vi "max XY speed.vi"() -> ()   [LabVIEW 2018]
uses:
  Classes/Controller/Controller.lvclass
  Drivers/Aerotech A3200/Aerotech.lvlib
panel:
  in  "stop":bool
  out "Y max speed":dbl
  out "X max speed":dbl
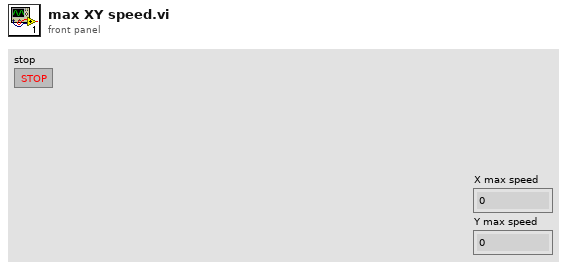
[diagram p1: front panel]
types:
  T1 = typedef "Controller.lvclass/Controllers.ctl" = cluster{"I-O.lvclass":refnum<class "I-O.lvclass">, "Gantry":refnum<k24>, "Dispenser":refnum<visa-resource-name>}
  T2 = typedef "Aerotech.lvlib/ControllerDiagPacket.ctl" = cluster{"Number of Diag Packets":i32, "Axes":T3[], "error":errorcluster}
  T3 = typedef "Aerotech.lvlib/AxisDiagPacket.ctl" = cluster{"Axis Name":string, "Analog Input 0":dbl, "Analog Input 1":dbl, "Axis Fault (num)":i32, "Axis Fault (str)":string, "Axis Fault (bits)":cluster{"AmplifierFault":bool, "AmplifierTemperatureFault":bool, "CcwEndOfTravelLimitFault":bool, "CcwSoftwareLimitFault":bool, "CommunicationLostFault":bool, "CwEndOfTravelLimitFault":bool, "CwSoftwareLimitFault":bool, "EmergencyStopFault":bool, "EncoderFault":bool, "ExternalFault":bool, "FeedbackScalingFault":bool, "GantryMisalignFault ":bool, "HallSensorFault":bool, "InPositionTimeoutFault":bool, "InternalFault":bool, "MarkerSearchFault":bool, "MaxVelocityCommandFault":bool, "MissedInterruptFault":bool, "MotorTemperatureFault":bool, "None":bool, "OverCurrentFault":bool, "PositionErrorFault":bool, "PositionFeedbackFault":bool, "PowerSupplyFault":bool, "ProbeInputFault":bool, "SafeZoneFault":bool, "VelocityErrorFault":bool, "VelocityFeedbackFault":bool, "VoltageClampFault":bool}, "Axis Status (num)":i32, "Axis Status (str)":string, "Axis Status (bits)":cluster{"BacklashActive":bool, "CalibrationEnabled1D":bool, "CalibrationEnabled2D":bool, "CommandValid":bool, "DriveAbortPending":bool, "DrivePending":bool, "Enabling":bool, "GainMappingEnabled":bool, "GantryAligned":bool, "GantryRealigning":bool, "Homed":bool, "Homing":bool, "IFOVEnabled":bool, "JogGenerating":bool, "Jogging":bool, "JoystickControl":bool, "MasterSlaveControl":bool, "MotionBlocked":bool, "MotionClamped":bool, "MoveDone":bool, "None":bool, "NotVirtual":bool, "Profiling":bool, "Stability0":bool, "Stability1":bool, "TrajectoryFiltering":bool, "WaitDone":bool}, "Current Command":sgl, "Current Error":sgl, "Current Feedback":sgl, "Digital Inputs":i32, "Digital Outputs":i32, "Drive Status":i32, "Drive Status (str)":string, "Drive Status (bits)":cluster{"AccelerationPhase":bool, "AutofocusActive":bool, "BrakeOutput":bool, "CcwEndOfTravelLimitInput":bool, "CosineEncoderError":bool, "CurrentClamp":bool, "CwEndOfTravelLimitInput":bool, "DecelerationPhase":bool, "DualLoopActive":bool, "EmergencyStopInput":bool, "Enabled":bool, "EncoderClipping":bool, "GalvoCalibrationEnabled":bool, "GalvoPowerCorrection":bool, "HallAInput":bool, "HallBInput":bool, "HallCInput":bool, "HighResolutionMode":bool, "HomeLimitInput":bool, "InPosition":bool, "InPosition2":bool, "MarkerInput":bool, "MarkerLatch":bool, "MoveActive":bool, "NoMotorSupply":bool, "None":bool, "PowerLimiting":bool, "ProgrammingFlash":bool, "ProgrammingMXH":bool, "PSOHaltLatch":bool, "ServoControl":bool, "SineEncoderError":bool}, "Position Feedback Auxiliary":dbl, "Position Command":dbl, "Position Error":dbl, "Position Feedback":dbl, "Program Position Command":dbl, "Program Position Error":dbl, "Program Position Feedback":dbl, "Velocity Command":dbl, "Velocity Error":dbl, "Velocity Feedback":dbl}
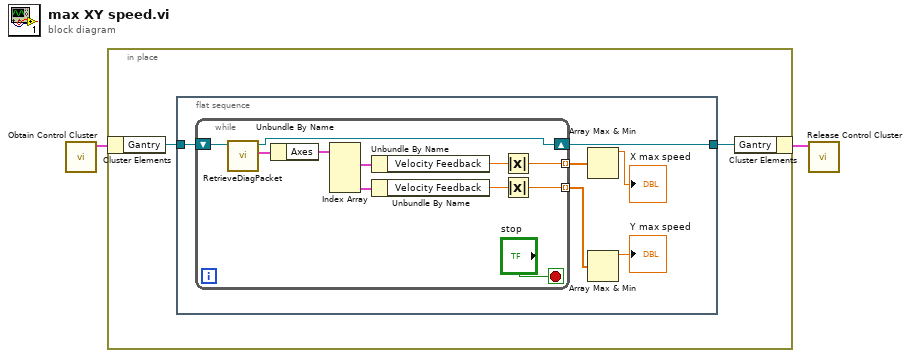
[diagram p0: block diagram]
diagram:
  n1 = call "Obtain Control Cluster.vi"() -> ("Control Out"=w2:T1)  [unwired: 11 in]
  n2 = in-place {
    n3 = in-place-cluster #1(w2) -> ("Gantry"=w4:refnum<k24>)
    n4 = flat-sequence {
      tunnel: w4 -> [w6]
      tunnel: [w5] -> w3
      frame #0 {
        n5 = while {
          tunnel: [w17] -> w7 mode=indexing
          tunnel: [w15] -> w8 mode=indexing
          shift-right: [w11] -> w5
          shift-left: w6 -> [w13]
          stop <- "stop" stop-if-true
          n6 = call "RetrieveDiagPacket.vi"("Controller In"=w13) -> ("ControllerDiagPacket"=w12:T2, "Controller Out"=w11:refnum<k24>)  [unwired: 8 in, 1 out]
          n7 = Unbundle By Name(w12) -> ("Axes"=w21:T3[])
          n8 = Index Array(array=w21) -> (element #1=w20:T3, element #4=w19:T3)  [unwired: 4 in, 2 out]
          n9 = Unbundle By Name(w20) -> ("Velocity Feedback"=w18:dbl)
          n10 = Unbundle By Name(w19) -> ("Velocity Feedback"=w16:dbl)
          n11 = Absolute Value(x=w18) -> (abs(x)=w17:dbl)
          n12 = Absolute Value(x=w16) -> (abs(x)=w15:dbl)
        }
        n13 = Array Max & Min(array=w7) -> (max value=→"X max speed":dbl)  [unwired: 3 out]
        n14 = Array Max & Min(array=w8) -> (max value=→"Y max speed":dbl)  [unwired: 3 out]
      }
    }
    n15 = in-place-cluster #1("Gantry"=w3) -> (w1:T1)
  }
  n16 = call "Release Control Cluster.vi"("output cluster"=w1) -> ()  [unwired: 11 in]
